vi "Microfone.vi"() -> ()   [LabVIEW 2014]
uses:
  <vilib>/myRIO/Instrument Drivers/Onboard IO/AI/typedefs/AI Reference.ctl
  <vilib>/myRIO/Common/Instrument Driver Framework/Utilities/typedefs/myRIO Generic Hardware Reference.ctl
  <vilib>/myRIO/Common/Instrument Driver Framework/Utilities/typedefs/Hardware Version Enum.ctl
  <vilib>/myRIO/Common/Instrument Driver Framework/Utilities/typedefs/myRIO v1.0 Reference.ctl
  <vilib>/myRIO/Common/Instrument Driver Framework/Utilities/typedefs/Generic FPGA Reference.ctl
  <vilib>/myRIO/Common/Instrument Driver Framework/myRIO v1.0/AI/typedefs/AI Channels List.ctl
  <vilib>/myRIO/Common/Instrument Driver Framework/myRIO v1.0/AI/typedefs/AI Channels Enum.ctl
  <vilib>/myRIO/Common/Instrument Driver Framework/Utilities/typedefs/Analog Scaling Constants List.ctl
  <vilib>/myRIO/Common/Instrument Driver Framework/Utilities/typedefs/Analog Scaling Constants.ctl
  <vilib>/userdefined/High Color/nirio_resource_hc.ctl
  <vilib>/myRIO/Common/Instrument Driver Framework/Utilities/vis/Is FPGA Ref Available.vi
  <vilib>/myRIO/Common/Instrument Driver Framework/myRIO v1.0/AI/vis/myRIO v1.1 Open AI.vi
  <vilib>/myRIO/Instrument Drivers/Onboard IO/AI/vis/Read.vi
  <vilib>/myRIO/Common/Instrument Driver Framework/Utilities/vis/Validate Channels.vi
  <vilib>/myRIO/Common/Instrument Driver Framework/myRIO v1.0/AI/vis/myRIO v1.0 Reserve AI.vi
  <vilib>/myRIO/Common/Instrument Driver Framework/myRIO v1.0/AI/vis/myRIO v1.0 Build MUX Configuration AI.vi
  <vilib>/myRIO/Common/Instrument Driver Framework/myRIO v1.0/Resource Manager/vis/myRIO v1.0 Reserve Channel List.vi
  <vilib>/myRIO/Common/Instrument Driver Framework/myRIO v1.0/Resource Manager/vis/myRIO v1.0 Reserve Channel.vi
  <vilib>/myRIO/Common/Instrument Driver Framework/myRIO v1.0/Resource Manager/vis/myRIO v1.0 Unreserve Channel.vi
  <vilib>/myRIO/Common/Instrument Driver Framework/myRIO v1.0/Resource Manager/vis/myRIO v1.0 Build Mutex Name.vi
  <vilib>/Utility/VariantDataType/GetNumericInfo.vi
  <vilib>/Utility/error.llb/Error Cluster From Error Code.vi
  <vilib>/myRIO/Common/Instrument Driver Framework/myRIO v1.0/myRIO v1.1 Open.vi
  <vilib>/myRIO/Common/Instrument Driver Framework/myRIO v1.0/AI/vis/myRIO v1.0 Get Scaling Constants AI.vi
  <vilib>/myRIO/Common/Instrument Driver Framework/Utilities/vis/IO Manager.vi
  <vilib>/myRIO/Common/Instrument Driver Framework/Utilities/vis/Configuration Manager.vi
  <vilib>/myRIO/Common/Instrument Driver Framework/myRIO v1.0/myRIO v1.0 Close.vi
  <vilib>/myRIO/Common/Instrument Driver Framework/myRIO v1.0/AI/vis/myRIO v1.0 Read AI.vi
  <vilib>/measure/matone.llb/Extract Multiple Tone Information N Chan.vi
  <vilib>/express/express analysis/Spectral/Block/exnSpectralBlock spectral measurements peak poly.vi
  <vilib>/express/express analysis/Spectral/Block/exnSpectralBlock spectral measurements peak DDT.vi
  <vilib>/myRIO/Express VI/Onboard IO/AI/AI Express VI.xnode
  <vilib>/myRIO/Instrument Drivers/Onboard IO/AI/vis/myRIO AI Open.xnode
  <vilib>/express/express analysis/Spectral/XNode/ExpressSpectralMeasurementsBlockNode.xnode
  <vilib>/measure/NI_MAPro.lvlib
  <vilib>/myRIO/Instrument Drivers/Onboard IO/AI/AI.lvlib
panel:
  out "formantes detectados":dbl[](array[numeric])
  out "U":bool
  out "O":bool
  out "A":bool
  in  "botão U":bool
  in  "botão O":bool
  out "O":dbl
  out "U":dbl
  out "A":dbl
  in  "botão A":bool
  out "XY Graph 2":cluster{"Array":cluster{"f1":dbl, "f2":dbl}[]}[](graph)
  out "Espectro de Amplitudes 2":waveform(dbl)(graph)
  in  "Threshold":dbl=0.001 format="%#_6p"
  out "multiple tone information":T1(array[cluster]) {"multiple tone information"."detected phase (deg)" format="%_6g"; "multiple tone information"."detected amplitude" format="%_6p"; "multiple tone information"."detected frequency" format="%_6p"}
  in  "Stop Button":bool
  out "Espectro de Amplitudes":dynamicdata(graph)
  out "Waveform Graph":dynamicdata(graph)
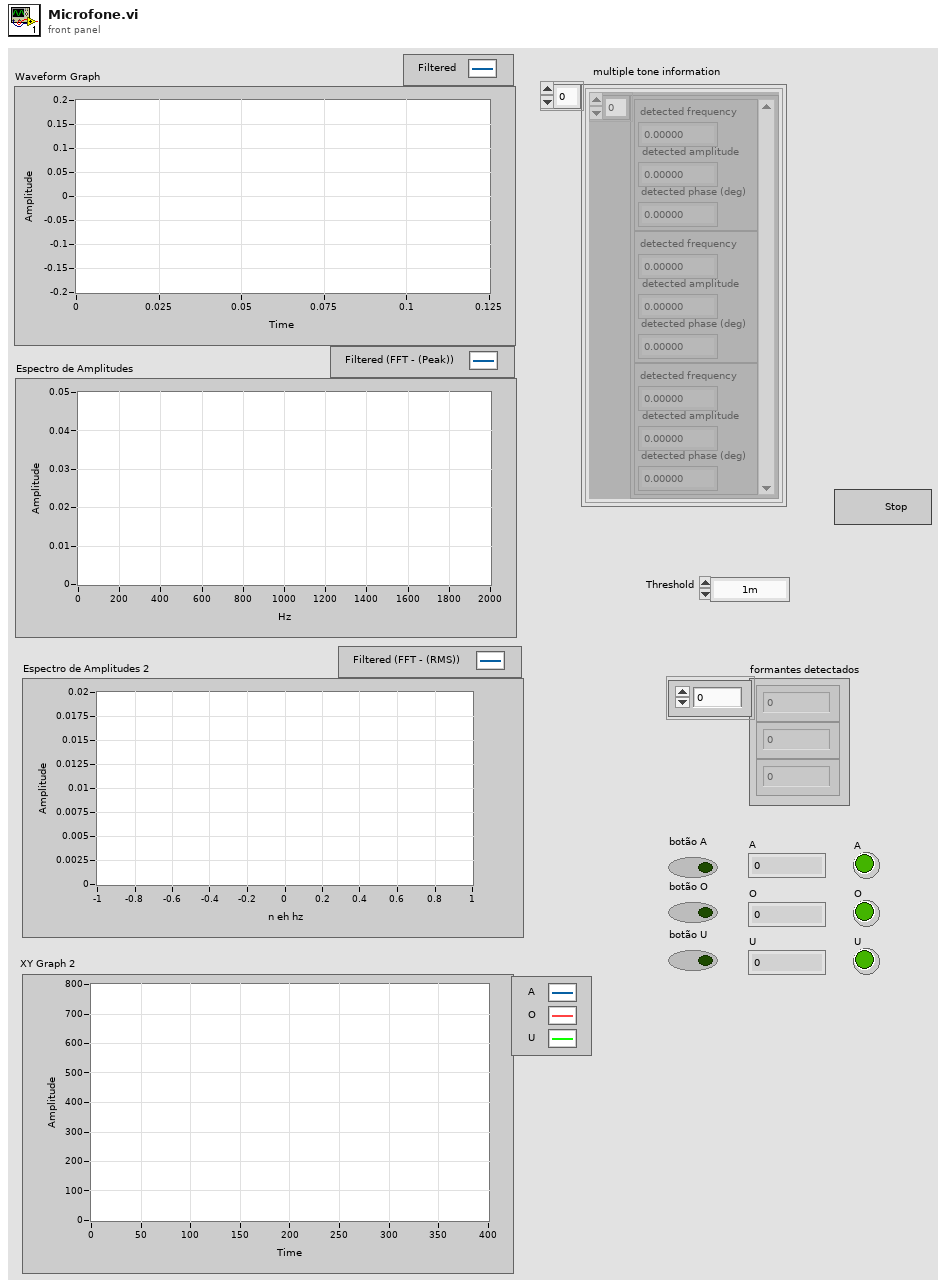
[diagram p1: front panel]
types:
  T1 = cluster{"multiple tone information":cluster{"detected frequency":dbl, "detected amplitude":dbl, "detected phase (deg)":dbl}[]}[]
  T2 = cluster{"averaging mode":u16, "weighting mode":u16, "number of averages":u32}
  T3 = cluster{"dB On (F)":bool, "unwrap phase (F)":bool, "convert to degree (F)":bool}
  T4 = typedef "AI.lvlib/AI Reference.ctl" = cluster{"myRIO Reference":T5, "AI Channels List":T9, "AI Scaling Constants List":T11}
  T5 = typedef "myRIO Generic Hardware Reference.ctl" = cluster{"myRIO Model":T6, "myRIO Hardware Reference":T7}
  T6 = typedef "Hardware Version Enum.ctl" = enum16{"Unknown", "myRIO-1900", "myRIO-1950"}
  T7 = typedef "myRIO v1.0 Reference.ctl" = cluster{"Generic FPGA Reference":T8, "Allow multiple opens":bool}
  T8 = typedef "Generic FPGA Reference.ctl" = refnum<k20>
  T9 = typedef "AI Channels List.ctl" = T10[]
  T10 = typedef "AI Channels Enum.ctl" = enum16{"Not Connected", "AudioIn/Left", "AudioIn/Right", "C/AI0", "C/AI1", "A/AI0", "A/AI1", "A/AI2", "A/AI3", "B/AI0", "B/AI1", "B/AI2", "B/AI3"}
  T11 = typedef "Analog Scaling Constants List.ctl" = T12[]
  T12 = typedef "Analog Scaling Constants.ctl" = cluster{"LSB Weight (Volts)":dbl, "Offset (Volts)":dbl, "Signed?":bool}
  T13 = typedef "nirio_resource_hc.ctl" = tag
  T14 = cluster{"multiple tone information":cluster{"detected frequency":dbl, "detected amplitude":dbl, "detected phase (deg)":dbl}[]}
  T15 = cluster{"detected frequency":dbl, "detected amplitude":dbl, "detected phase (deg)":dbl}[]
  T16 = cluster{"detected frequency":dbl, "detected amplitude":dbl, "detected phase (deg)":dbl}
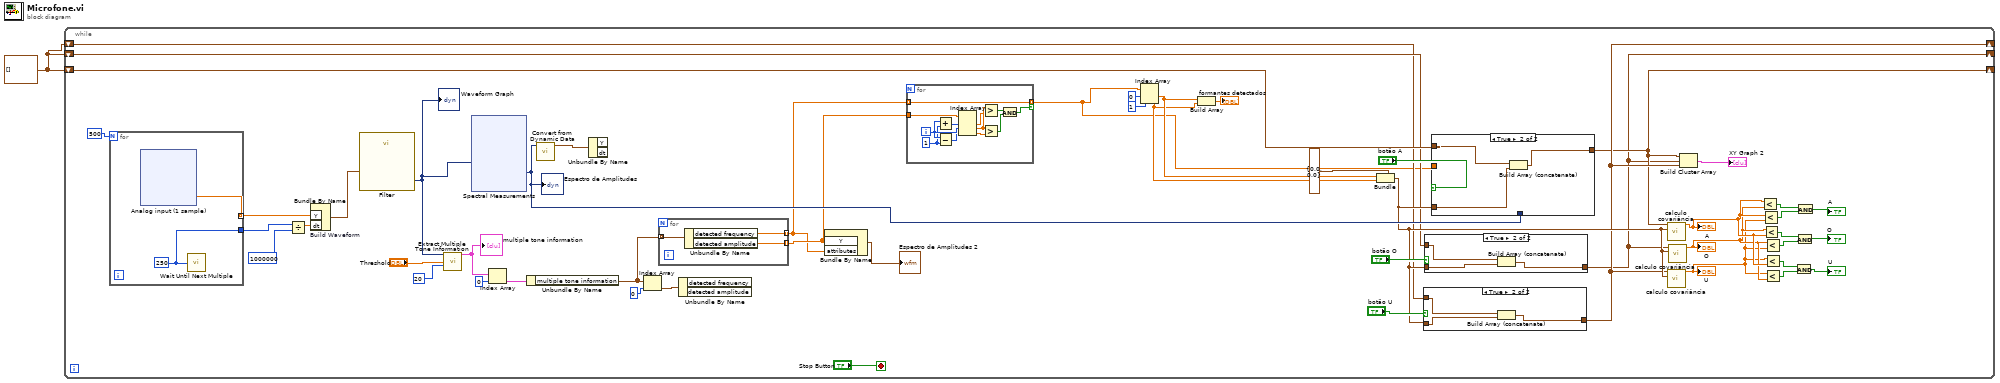
[diagram p0: block diagram]
diagram:
  w1 = cluster{"f1":dbl, "f2":dbl}[] [] ("Array")
  n1 = while {
    shift-right: [w8] -> _
    shift-left: w1 -> [w23]
    shift-right: [w7] -> _
    shift-left: w1 -> [w21]
    shift-right: [w19] -> _
    shift-left: w1 -> [w20]
    stop <- "Stop Button" stop-if-true
    n2 = for {
      N: 500 -> [_]
      tunnel: [w91] -> w50 mode=indexing
      tunnel: [w90] -> w49
      w90 = u32 250 ("Count(uSec)")
      n3 = xnode "Analog input (1 sample)"() -> ("AudioIn/Left"=w91:dbl)  [unwired: 1 in, 1 out]
      n4 = call "Wait Until Next Multiple"("Count(uSec)"=w90) -> ()  [unwired: 1 out]
    }
    n5 = Divide(x=w49, y=u32 1000000) -> (x/y=w48:dbl)
    n6 = Bundle By Name "Build Waveform"("Y"=w50, "dt"=w48) -> (w46:waveform(dbl))  [unwired: 1 in]
    n7 = call "Filter"("Signal"=w46) -> ("Filtered Signal"=w45:dynamicdata)  [unwired: 9 in, 1 out]
    "Waveform Graph" <- w45
    n8 = call-poly <vilib>:"Extract Multiple Tone Information.vi"("time signals in"=w45, "threshold"="Threshold", "max num tones"=20) -> ("multiple tone information"=w44:T1)  [unwired: 10 in, 2 out]
    "multiple tone information" <- w44
    n9 = xnode "Spectral Measurements"("Signals"=w45) -> ("FFT - (Peak)"=w33:dynamicdata)  [unwired: 1 in, 2 out]
    "Espectro de Amplitudes" <- w33
    n10 = Index Array(array=w44, index=0) -> (element=w42:T14)
    n11 = Unbundle By Name(w42) -> ("multiple tone information"=w36:T15)
    n12 = call "Convert from Dynamic Data"("Dynamic Data Type"=w33) -> ("Waveform"=w37:waveform(dbl))  [unwired: 3 in]
    n13 = Unbundle By Name(w37) -> ()  [unwired: 2 out]
    n14 = Index Array(array=w36, index=0) -> (element=w40:T16)
    n15 = for {
      tunnel: w36 -> [w79] mode=indexing
      tunnel: [w78] -> w31 mode=indexing
      tunnel: [w77] -> w32 mode=indexing
      n16 = Unbundle By Name(w79) -> ("detected frequency"=w78:dbl, "detected amplitude"=w77:dbl)
    }
    n17 = Unbundle By Name(w40) -> ()  [unwired: 2 out]
    n18 = Bundle By Name("Y"=w32, "attributes"=w31) -> (→"Espectro de Amplitudes 2":waveform(dbl))  [unwired: 1 in]
    n19 = for {
      tunnel: w32 -> [w76]
      tunnel: [w65] -> w18 mode=indexing if=w66
      tunnel: w31 -> [w65] mode=indexing
      i -> [w75]
      w74 = 1 ("y")
      n20 = Add(x=w75, y=w74) -> (x+y=w73:i32)
      n21 = Subtract(x=w75, y=w74) -> (x-y=w72:i32)
      n22 = Index Array(array=w76, index #1=w73, index #2=w75, index #3=w72) -> (element #1=w67:dbl, element #2=w71:dbl, element #3=w70:dbl)
      n23 = Greater?(x=w71, y=w67) -> (0:w69:bool)
      n24 = Greater?(x=w71, y=w70) -> (0:w68:bool)
      n25 = And(x=w69, y=w68) -> (x .and. y?=w66:bool)
    }
    n26 = Index Array(array=w18, index #1=0 ("index"), index #2=1 ("index")) -> (element #1=w28:dbl, element #2=w27:dbl)
    n27 = Build Array(w28, w27) -> (→"formantes detectados":dbl[])
    n28 = Bundle(cluster=cluster{"f1":dbl, "f2":dbl} {"f1"=0.0, "f2"=0.0}, "f1"=w28, "f2"=w27) -> (w22:cluster{"f1":dbl, "f2":dbl})
    n29 = case shown="True" "botão U" {
      tunnel: [w53 w56] -> w19
      tunnel: w22 -> [_ w55]
      tunnel: w20 -> [w53 w54]
      frame False {
      }
      frame True {
        n30 = Build Array (concatenate)(w54, w55) -> (w56:cluster{"f1":dbl, "f2":dbl}[])
      }
    }
    n31 = case shown="True" "botão O" {
      tunnel: w22 -> [_ w60]
      tunnel: [w57 w59] -> w7
      tunnel: w21 -> [w57 w58]
      frame False {
      }
      frame True {
        n32 = Build Array (concatenate)(w58, w60) -> (w59:cluster{"f1":dbl, "f2":dbl}[])
      }
    }
    n33 = case shown="True" "botão A" {
      tunnel: w22 -> [_ w64]
      tunnel: [w61 w62] -> w8
      tunnel: w23 -> [w61 w63]
      tunnel: w33 -> [_ _]
      tunnel: w18 -> [_ _]
      frame False {
      }
      frame True {
        n34 = Build Array (concatenate)(w63, w64) -> (w62:cluster{"f1":dbl, "f2":dbl}[])
      }
    }
    n35 = call "calculo covariância.vi"("cluster"=w22, "Array"=w8) -> ("element"=w4:dbl)  [unwired: 9 in]
    "A" <- w4
    n36 = call "calculo covariância.vi"("cluster"=w22, "Array"=w19) -> ("element"=w2:dbl)  [unwired: 9 in]
    "U" <- w2
    n37 = call "calculo covariância.vi"("cluster"=w22, "Array"=w7) -> ("element"=w3:dbl)  [unwired: 9 in]
    "O" <- w3
    n38 = Build Cluster Array(w8, w7, w19) -> (→"XY Graph 2":cluster{"Array":cluster{"f1":dbl, "f2":dbl}[]}[])
    n39 = Less?(x=w4, y=w3) -> (x < y?=w16:bool)
    n40 = Less?(x=w4, y=w2) -> (x < y?=w15:bool)
    n41 = Less?(x=w3, y=w4) -> (x < y?=w14:bool)
    n42 = Less?(x=w3, y=w2) -> (x < y?=w13:bool)
    n43 = Less?(x=w2, y=w4) -> (x < y?=w12:bool)
    n44 = Less?(x=w2, y=w3) -> (x < y?=w11:bool)
    n45 = And(x=w12, y=w11) -> (x .and. y?=→"U":bool)
    n46 = And(x=w14, y=w13) -> (x .and. y?=→"O":bool)
    n47 = And(x=w16, y=w15) -> (x .and. y?=→"A":bool)
  }
